vi "Process New Connection.vi"(8 "error in (no error)":errorcluster, 10 "Connection Reference":refnum<data-value>, 11 "MultiplexedConnectionHandler in":refnum<class "MultiplexedConnectionHandler.lvclass">) -> (0 "error out":errorcluster, 3 "MultiplexedConnectionHandler out":refnum<class "MultiplexedConnectionHandler.lvclass">)   [LabVIEW 2020, in "MultiplexedConnectionHandler.lvlib" / "MultiplexedConnectionHandler.lvclass"]
uses:
  <vilib>/gpm_packages/@cs/Network-interface/Source/MultiplexedConnectionHandler/MultiplexedConnectionHandler/MultiplexedConnectionHandler.lvclass
  C:/Program Files/National Instruments/LabVIEW 2020/vi.lib/gpm_packages/@cs/Network-interface/Source/PersistantConnectionHandler/PersistantConnectionHandler/PersistantConnectionHandler.lvclass
  <vilib>/gpm_packages/@cs/Network-interface/Source/Connection Reference/Connection Reference/Connection Reference.lvclass
  <vilib>/gpm_packages/@cs/Network-interface/Source/MultiplexedConnectionHandler/MultiplexedConnectionHandler/MultiplexedConnectionHandler.lvclass/MultiplexedConnectionHandler.ctl
  <vilib>/gpm_packages/@cs/Network-interface/Source/PersistantConnectionHandler/PersistantConnectionHandler/PersistantConnectionHandler.lvclass
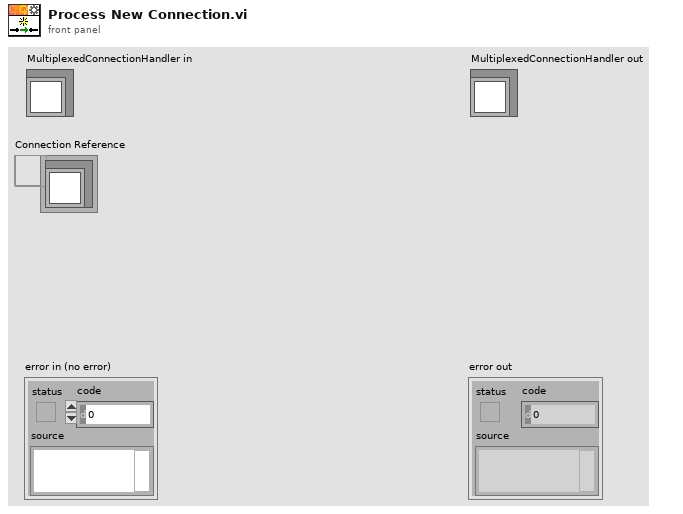
[diagram p1: front panel]
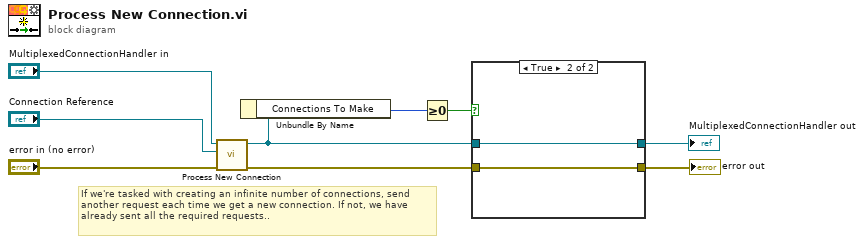
[diagram p0: block diagram]
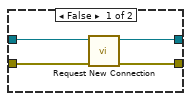
[diagram p2: hidden frame]
diagram:
  # "If we're tasked with creating an infinite number of connections, send another request each time we get a new connection. If not, we have already sent all the required requests.."
  n1 = call-parent "Process New Connection.vi"("error in (no error)"="error in (no error)", "Connection Reference"="Connection Reference", "PersistantConnectionHandler in"="MultiplexedConnectionHandler in") -> ("error out"=w6:errorcluster, "PersistantConnectionHandler out"=w3:refnum<class "MultiplexedConnectionHandler.lvclass">)  [unwired: 7 in]
  n2 = Unbundle By Name(w3) -> ("Connections To Make"=w2:i32)
  n3 = Greater Or Equal To 0?(x=w2) -> (x >= 0?=w1:bool)
  n4 = case shown="True" w1 {
    tunnel: w3 -> [w13 w15]
    tunnel: w6 -> [w12 w14]
    tunnel: [w11 w15] -> w5
    tunnel: [w10 w14] -> w4
    frame False {
      n5 = call <vilib>:"Request New Connection.vi"("error in (no error)"=w12, "PersistantConnectionHandler in"=w13) -> ("error out"=w10:errorcluster, "PersistantConnectionHandler out"=w11:refnum<class "MultiplexedConnectionHandler.lvclass">)  [unwired: 8 in]
    }
    frame True {
    }
  }
  "error out" <- w4
  "MultiplexedConnectionHandler out" <- w5
